vi "setUp.vi"(8 "error in (no error)":errorcluster, 11 "reference in":refnum<class "Logging Loopback.lvclass">) -> (0 "error out":errorcluster, 3 "reference out":refnum<class "Logging Loopback.lvclass">)   [LabVIEW 2020, in "Logging Loopback.lvclass"]
doc: "setUp runs prior to the test method during test execution. Use this method to initialize any object data required by your tests."
uses:
  Logging Loopback.lvclass
  <vilib>/addons/_JKI Toolkits/VI Tester/TestCase.llb/TestCase.lvclass
  niveristand-custom-device-testing-tools/VeriStandTestUtilities/VeriStandTestUtilities.lvlib
  <vilib>/WebDAVClient/NI_WebDAV.lvlib
  C:/Program Files (x86)/National Instruments/LabVIEW 2020/vi.lib/addons/_JKI Toolkits/VI Tester/TestCase.llb/TestCase.lvclass
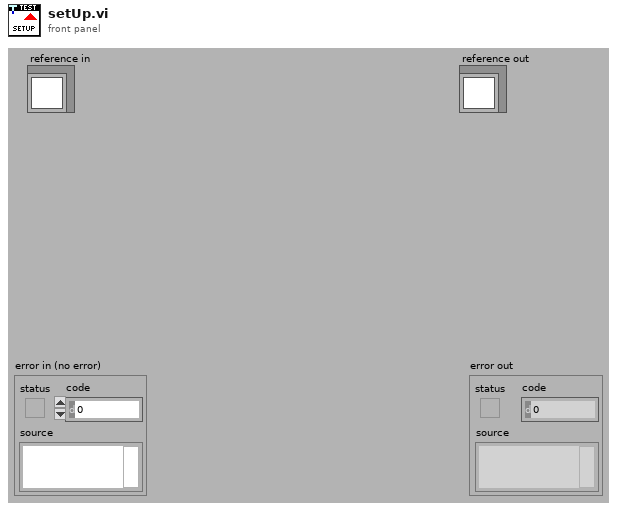
[diagram p1: front panel]
types:
  T1 = typedef "Custom Device API.lvlib/Custom Device Item Ref.ctl" = u64
  T2 = typedef "NI_WebDAV.lvlib/SessionHandle.ctl" = refnum<k1>
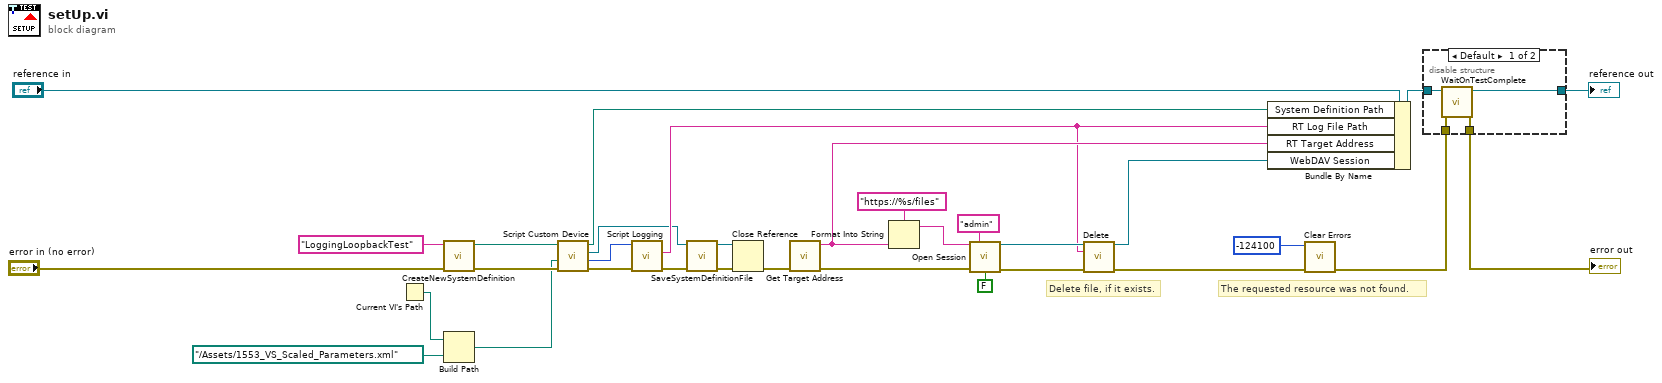
[diagram p0: block diagram]
diagram:
  # "Delete file, if it exists."
  # "The requested resource was not found."
  n1 = Current VI's Path() -> (path=w1:path)
  n2 = call "CreateNewSystemDefinition.vi"("error in"="error in (no error)", "System Definition Name"="LoggingLoopbackTest" ("Channel")) -> ("error out"=w10:errorcluster, "System Definition Path"=w9:path)  [unwired: 8 in]
  n3 = Build Path(base path=w1, name or relative path=path "../Assets/1553_VS_Scaled_Parameters.xml" ("Hardware File Path")) -> (appended path=w2:path)
  n4 = call "Script Custom Device.vi"("error in"=w10, "parameters configuration file path"=w2, "system definition path in"=w9) -> ("error out"=w7:errorcluster, "AIM MIL-STD 1553 custom device out"=w6:T1, "System Definition"=w8:refnum<k24>, "system definition path out"=w15:path)  [unwired: 5 in]
  n5 = call "Script Logging.vi"("error in (no error)"=w7, "Ballard MIL-STD 1553 custom device in"=w6) -> ("error out"=w5:errorcluster, "RT log file path"=w19:string)  [unwired: 7 in, 1 out]
  n6 = call "SaveSystemDefinitionFile.vi"("error in (no error)"=w5, "System Definition Reference in"=w8) -> ("error out"=w4:errorcluster, "System Definition Reference out"=w3:refnum<k24>)  [unwired: 8 in]
  n7 = Close Reference(reference=w3, error in (no error)=w4) -> (error out=w27:errorcluster)
  n8 = call "Get Target Address.vi"("error in (no error)"=w27) -> ("error out"=w21:errorcluster, "target address"=w20:string)  [unwired: 9 in]
  n9 = Format Into String(format string="https://%s/files" ("host uri prefix"), w20) -> (resulting string=w22:string)  [unwired: 2 in, 1 out]
  n10 = call <vilib>:"Open Session.vi"("host uri prefix"=w22, "username"="admin", "error in (no error)"=w21, "verify server?"=FALSE) -> ("session handle out"=w26:T2, "error out"=w25:errorcluster)  [unwired: 10 in]
  n11 = call <vilib>:"Delete.vi"("session handle"=w26, "relative uri"=w19, "error in (no error)"=w25) -> ("session handle out"=w13:T2, "error out"=w17:errorcluster)  [unwired: 11 in]
  n12 = Bundle By Name(cluster="reference in", "System Definition Path"=w15, "RT Log File Path"=w19, "RT Target Address"=w20, "WebDAV Session"=w13) -> (w28:refnum<class "Logging Loopback.lvclass">)
  n13 = call <vilib>:"Clear Errors.vi"("error in (no error)"=w17, "specific error code to clear (0: all)"=-124100) -> ("error out"=w14:errorcluster)  [unwired: 4 in, 1 out]
  n14 = disable-structure shown="Default" {
    disable-tunnel: w14 -> [w36 w37]
    disable-tunnel: [w35 w37] -> w32
    disable-tunnel: [w34 w38] -> w30
    disable-tunnel: w28 -> [w33 w38]
    frame condition #0 (active) {
      n15 = call <vilib>:"WaitOnTestComplete.vi"("error in (no error)"=w36, "TestCase in"=w33) -> ("error out"=w35:errorcluster, "TestCase out"=w34:refnum<class "Logging Loopback.lvclass">)  [unwired: 8 in]
    }
    frame condition #1 {
    }
  }
  "error out" <- w32
  "reference out" <- w30
